vi "Read Status.vi"(8 "error in (no error)":errorcluster, 11 "Image Processing Handler in":refnum<class "Image Processing Handler.lvclass">) -> (0 "error out":errorcluster, 2 "Status":T1, 3 "Image Processing Handler out":refnum<class "Image Processing Handler.lvclass">)   [LabVIEW 2018, in "Image Processing Handler.lvclass"]
uses:
  Image Processing Handler.lvclass
  Video Frame/Video Frame.lvclass
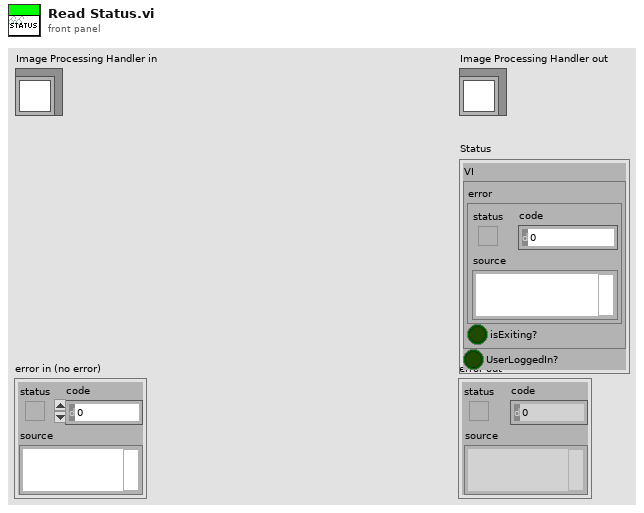
[diagram p1: front panel]
types:
  T1 = cluster{"VI":cluster{"error":errorcluster, "isExiting?":bool}, "UserLoggedIn?":bool}
  T2 = cluster{"VI":cluster{"error":errorcluster, "isExiting?":bool}, "UserLoggedIn?":bool, "Video Frame":refnum<class "Video Frame.lvclass">}
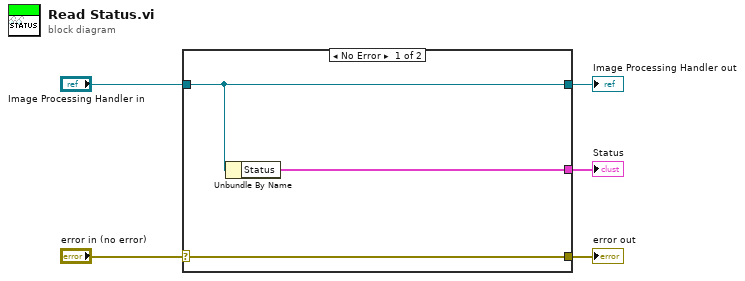
[diagram p0: block diagram]
diagram:
  n1 = case shown="No Error" "error in (no error)" {
    selector: "error in (no error)" -> [w8 w9]
    tunnel: [w8 w9] -> w4
    tunnel: [w7 w10] -> w2
    tunnel: "Image Processing Handler in" -> [w7 w10]
    tunnel: [w6 _] -> w1
    frame No Error {
      n2 = Unbundle By Name(w7) -> ("Status"=w6:T2)
    }
    frame Error {
    }
  }
  "error out" <- w4
  "Image Processing Handler out" <- w2
  "Status" <- w1
